vi "Main - UDP.vi"() -> ()   [LabVIEW 2023]
uses:
  <vilib>/addons/VeriStand Custom Device Scripting APIs/Data Sharing Framework/DSF Core.lvlibp/Typedefs/DSF Engine Framework Configuration.ctl
  <vilib>/addons/VeriStand Custom Device Scripting APIs/Data Sharing Framework/DSF Core.lvlibp/Typedefs/DSF Engine Plugin Configuration.ctl
  <vilib>/addons/VeriStand Custom Device Scripting APIs/Data Sharing Framework/DSF Core.lvlibp/Typedefs/Core Plugin Configuration.ctl
  <vilib>/addons/VeriStand Custom Device Scripting APIs/Data Sharing Framework/DSF Core.lvlibp/Typedefs/DSF Timing Info.ctl
  <vilib>/addons/VeriStand Custom Device Scripting APIs/Data Sharing Framework/DSF Core.lvlibp/Typedefs/DSF Settings Info.ctl
  <vilib>/addons/VeriStand Custom Device Scripting APIs/Data Sharing Framework/DSF Core.lvlibp/Typedefs/DSF Engine Plugin Thread Configuration.ctl
  <vilib>/addons/VeriStand Custom Device Scripting APIs/Data Sharing Framework/DSF Core.lvlibp/Typedefs/Core Thread Configuration.ctl
  <vilib>/addons/VeriStand Custom Device Scripting APIs/Data Sharing Framework/DSF Core.lvlibp/Typedefs/DSF Engine Transfer Group Configuration.ctl
  <vilib>/addons/VeriStand Custom Device Scripting APIs/Data Sharing Framework/DSF Core.lvlibp/Typedefs/Core Group Configuration.ctl
  <vilib>/addons/VeriStand Custom Device Scripting APIs/Data Sharing Framework/DSF Core.lvlibp/Typedefs/DSF Direction.ctl
  <vilib>/addons/VeriStand Custom Device Scripting APIs/Data Sharing Framework/DSF Core.lvlibp/Typedefs/DSF Timeout Behavior.ctl
  <vilib>/addons/VeriStand Custom Device Scripting APIs/Data Sharing Framework/DSF Core.lvlibp/Typedefs/DSF Engine Transfer Configuration.ctl
  <vilib>/addons/VeriStand Custom Device Scripting APIs/Data Sharing Framework/DSF Core.lvlibp/Typedefs/Core Transfer Configuration.ctl
  <vilib>/addons/VeriStand Custom Device Scripting APIs/Data Sharing Framework/DSF Core.lvlibp/Typedefs/DSF Engine Channel Configuration.ctl
  <vilib>/addons/VeriStand Custom Device Scripting APIs/Data Sharing Framework/DSF Core.lvlibp/Typedefs/Core Channel Configuration.ctl
  <vilib>/addons/VeriStand Custom Device Scripting APIs/Data Sharing Framework/DSF Core.lvlibp/Typedefs/DSF Data Type.ctl
  <userlib>/_OpenG.lib/array/array.llb/Index 1D Array Elements (String)__ogtk.vi
  <userlib>/_OpenG.lib/array/array.llb/Remove Duplicates from 1D Array (String)__ogtk.vi
  <userlib>/_OpenG.lib/array/array.llb/Filter 1D Array with Scalar (String)__ogtk.vi
  <vilib>/addons/VeriStand Custom Device Scripting APIs/Data Sharing Framework/DSF Core.lvlibp
  <vilib>/addons/VeriStand Custom Device Scripting APIs/Data Sharing Framework/DSF Core.lvlibp/Classes/Configuration/Core/Channel/Channel Configuration.lvclass
  <userlib>/_OpenG.lib/array/array.llb/openg_array.lvlib
  <vilib>/addons/VeriStand Custom Device Scripting APIs/Data Sharing Framework/DSF Core.lvlibp/Classes/Configuration/Core/Plugin/Plugin Configuration.lvclass
  <vilib>/addons/VeriStand Custom Device Scripting APIs/Data Sharing Framework/DSF Core.lvlibp/Classes/Configuration/Core/Thread/Thread Configuration.lvclass
  <vilib>/addons/VeriStand Custom Device Scripting APIs/Data Sharing Framework/DSF Core.lvlibp/Classes/Configuration/Core/Group/Group Configuration.lvclass
  <vilib>/addons/VeriStand Custom Device Scripting APIs/Data Sharing Framework/DSF Core.lvlibp/Classes/Configuration/Core/Transfer/Transfer Configuration.lvclass
panel:
  in  "Tab Control":enum32{"Main", "Raw Data", "Raw JSON"}(tab)
  out "DSF Clusters":T1[](array[typedef])
  out "Target Sources":string[](array[string])
  out "Channel Names":string[](array[string])
  out "Channel Units":string[](array[string])
  out "Channel Types":string[](array[string])
  out "Target Destinations":string[][](array[string])
  out "JSON Strings":string[](array[string])
  out "IP Addresses":string[](array[string])
  out "Target Names":string[](array[string])
  in  "File Path Control":path
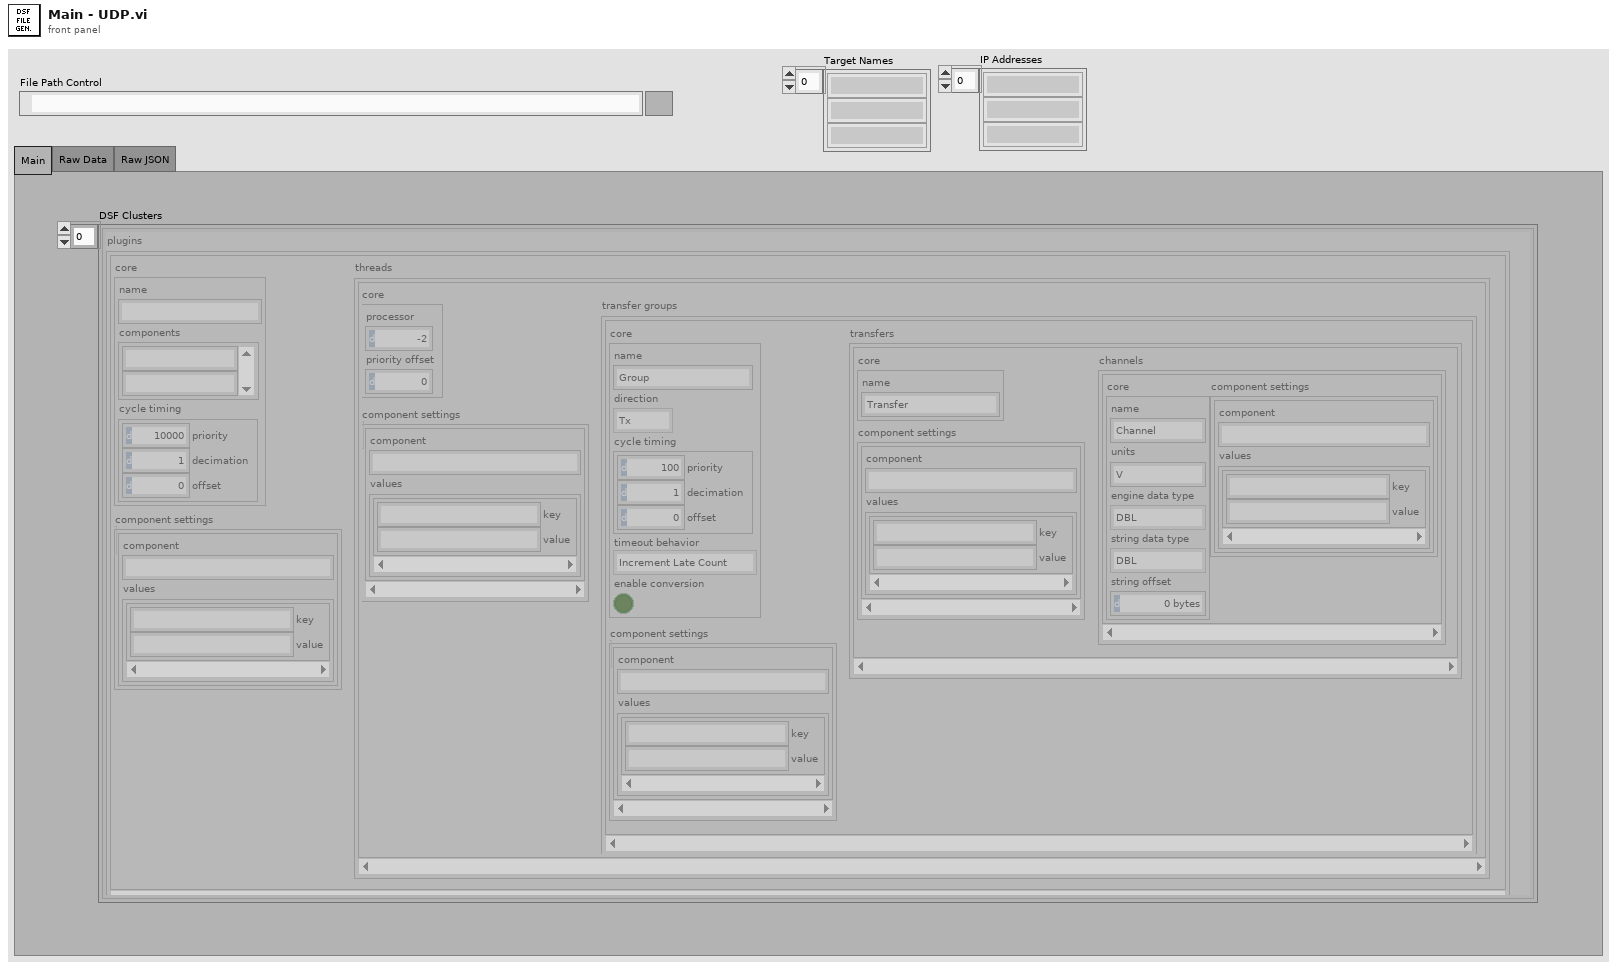
[diagram p1: front panel]
types:
  T1 = typedef "DSF Core.lvlibp/DSF Engine Framework Configuration.ctl" = cluster{"plugins":T2[]}
  T2 = typedef "DSF Core.lvlibp/DSF Engine Plugin Configuration.ctl" = cluster{"core":T3, "component settings":T5[], "threads":T6[]}
  T3 = typedef "DSF Core.lvlibp/Plugin Configuration.lvclass/Core Plugin Configuration.ctl" = cluster{"name":string, "components":string[], "cycle timing":T4}
  T4 = typedef "DSF Core.lvlibp/DSF Timing Info.ctl" = cluster{"priority":u64, "decimation":u64, "offset":u64}
  T5 = typedef "DSF Core.lvlibp/DSF Settings Info.ctl" = cluster{"component":string, "values":cluster{"key":string, "value":string}[]}
  T6 = typedef "DSF Core.lvlibp/DSF Engine Plugin Thread Configuration.ctl" = cluster{"core":T7, "component settings":T5[], "transfer groups":T8[]}
  T7 = typedef "DSF Core.lvlibp/Thread Configuration.lvclass/Core Thread Configuration.ctl" = cluster{"processor":i32, "priority offset":i16}
  T8 = typedef "DSF Core.lvlibp/DSF Engine Transfer Group Configuration.ctl" = cluster{"core":T9, "component settings":T5[], "transfers":T12[]}
  T9 = typedef "DSF Core.lvlibp/Group Configuration.lvclass/Core Group Configuration.ctl" = cluster{"name":string, "direction":T10, "cycle timing":T4, "timeout behavior":T11, "enable conversion":bool}
  T10 = typedef "DSF Core.lvlibp/DSF Direction.ctl" = enum8{"Tx", "Rx"}
  T11 = typedef "DSF Core.lvlibp/DSF Timeout Behavior.ctl" = enum8{"Increment Late Count", "Throw Error"}
  T12 = typedef "DSF Core.lvlibp/DSF Engine Transfer Configuration.ctl" = cluster{"core":T13, "component settings":T5[], "channels":T14[]}
  T13 = typedef "DSF Core.lvlibp/Transfer Configuration.lvclass/Core Transfer Configuration.ctl" = cluster{"name":string}
  T14 = typedef "DSF Core.lvlibp/DSF Engine Channel Configuration.ctl" = cluster{"core":T15, "component settings":T5[]}
  T15 = typedef "DSF Core.lvlibp/Channel Configuration.lvclass/Core Channel Configuration.ctl" = cluster{"name":string, "units":string, "engine data type":T16, "string data type":T16, "string offset":u64}
  T16 = typedef "DSF Core.lvlibp/DSF Data Type.ctl" = enum8{"Bool", "SGL", "DBL", "I8", "I16", "I32", "I64", "U8", "U16", "U32", "U64"}
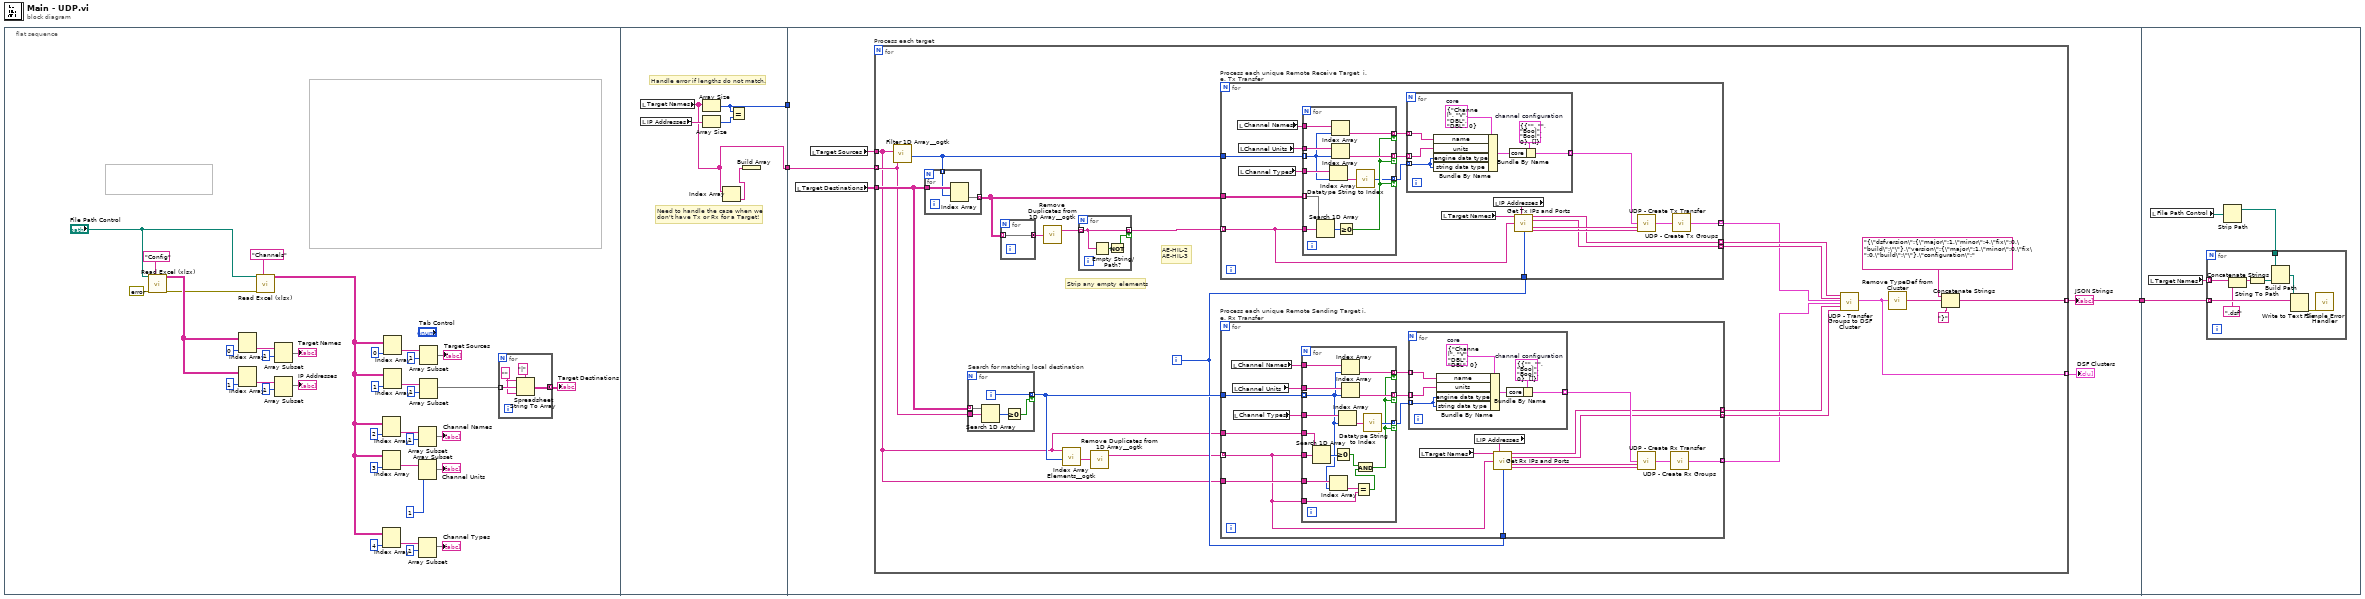
[diagram p0: block diagram]
diagram:
  n1 = flat-sequence {
    tunnel: [w47] -> w3
    tunnel: [w44] -> w1
    tunnel: w3 -> [_]
    tunnel: [w49] -> w2
    tunnel: w1 -> [w53]
    tunnel: w2 -> [w173]
    frame #0 {
      n2 = call "Read Excel (xlsx).vi"("Excel._SheetName"="Config", "error in (no error)"=errorcluster {"status"=FALSE, "code"=0, "source"=""}, "File Path Control"="File Path Control") -> ("error out"=w9:errorcluster, "data"=w10:string[][])  [unwired: 7 in]
      n3 = Index Array(array=w10, index (col)=0 ("disabled index (col)")) -> (element=w37:string[])  [unwired: 1 in]
      n4 = Index Array(array=w10, index (col)=1 ("disabled index (col)")) -> (element=w33:string[])  [unwired: 1 in]
      n5 = call "Read Excel (xlsx).vi"("Excel._SheetName"="Channels", "error in (no error)"=w9, "File Path Control"="File Path Control") -> ("data"=w8:string[][])  [unwired: 7 in, 1 out]
      n6 = Array Subset(array=w37, index=1) -> (→"Target Names":string[])  [unwired: 1 in]
      n7 = Array Subset(array=w33, index=1) -> (→"IP Addresses":string[])  [unwired: 1 in]
      n8 = Index Array(array=w8, index (col)=2 ("disabled index (col)")) -> (element=w22:string[])  [unwired: 1 in]
      n9 = Index Array(array=w8, index (col)=3 ("disabled index (col)")) -> (element=w18:string[])  [unwired: 1 in]
      n10 = Index Array(array=w8, index (col)=4 ("disabled index (col)")) -> (element=w14:string[])  [unwired: 1 in]
      n11 = Index Array(array=w8, index (col)=0 ("disabled index (col)")) -> (element=w29:string[])  [unwired: 1 in]
      n12 = Index Array(array=w8, index (col)=1 ("disabled index (col)")) -> (element=w25:string[])  [unwired: 1 in]
      n13 = Array Subset(array=w22, index=1) -> (→"Channel Names":string[])  [unwired: 1 in]
      n14 = Array Subset(array=w18, index=1) -> (→"Channel Units":string[])  [unwired: 1 in]
      n15 = Array Subset(array=w14, index=1) -> (→"Channel Types":string[])  [unwired: 1 in]
      n16 = Array Subset(array=w29, index=1) -> (→"Target Sources":string[])  [unwired: 1 in]
      n17 = Array Subset(array=w25, index=1) -> (w5:string[])  [unwired: 1 in]
      n18 = for {
        tunnel: w5 -> [w43] mode=indexing
        tunnel: [w41] -> w4 mode=concatenating
        w40 = ""
        n19 = Spreadsheet String To Array(delimiter (Tab)="|", format string=w40, spreadsheet string=w43, array type (2D Dbl)=w40) -> (array=w41:string[][])
      }
      "Target Destinations" <- w4
    }
    frame #1 {
      # "Need to handle the case when we \ndon't have Tx or Rx for a Target!"
      # "Handle error if lengths do not match."
      n20 = local read "Target Names"() -> (w44:string[])
      n21 = local read "IP Addresses"() -> (w46:string[])
      n22 = Array Size(array=w44) -> (size(s)=w47:i32)
      n23 = Array Size(array=w46) -> (size(s)=w48:i32)
      n24 = Index Array(array=w44) -> (element=w45:string)  [unwired: 1 in]
      n25 = Equal?(x=w47, y=w48) -> ()  [unwired: 1 out]
      n26 = Build Array(w45) -> ()  [unwired: 1 out]
    }
    frame #2 {
      n27 = local read "Target Destinations"() -> (w51:string[][])
      n28 = local read "Target Sources"() -> (w52:string[])
      n29 = for "Process each target" {
        tunnel: w53 -> [w61] mode=indexing
        tunnel: w52 -> [w60]
        tunnel: w51 -> [w70]
        tunnel: [w64] -> w49 mode=indexing
        tunnel: [w63] -> w50 mode=indexing
        i -> [w68]
        # "AE-HIL-2\nAE-HIL-3"
        # "Strip any empty elements"
        n30 = call-poly <userlib>:"Filter 1D Array__ogtk.vi"("items to filter"=w61, "array"=w60) -> ("filtered item indices"=w73:i32[])  [unwired: 4 in, 1 out]
        n31 = for {
          tunnel: w73 -> [w169] mode=indexing
          tunnel: w70 -> [w170]
          tunnel: [w168] -> w72 mode=indexing
          n32 = Index Array(array=w170, index (row)=w169) -> (element=w168:string[])  [unwired: 1 in]
        }
        n33 = for "Search for matching local destination" {
          tunnel: w70 -> [w125] mode=indexing
          tunnel: w61 -> [w124]
          tunnel: [w122] -> w69 mode=indexing if=w121
          i -> [w122]
          n34 = Search 1D Array(1D array=w125, element=w124) -> (index of element=w123:i32)  [unwired: 1 in]
          n35 = Greater Or Equal To 0?(x=w123) -> (x >= 0?=w121:bool)
        }
        n36 = for {
          tunnel: w72 -> [w167] mode=indexing
          tunnel: [w167] -> w76 mode=concatenating
        }
        n37 = call-poly <userlib>:"Remove Duplicates from 1D Array__ogtk.vi"("Input Array"=w76) -> ("Output Array"=w75:string[])  [unwired: 1 out]
        n38 = call-poly <userlib>:"Index Array Elements__ogtk.vi"("indices"=w69, "array"=w60) -> ("elements"=w71:string[])  [unwired: 9 in]
        n39 = for {
          tunnel: w75 -> [w166] mode=indexing
          tunnel: [w166] -> w74 mode=indexing if=w164
          n40 = Empty String/Path?(string/path=w166) -> (empty?=w165:bool)
          n41 = Not(x=w165) -> (.not. x?=w164:bool)
        }
        n42 = call-poly <userlib>:"Remove Duplicates from 1D Array__ogtk.vi"("Input Array"=w71) -> ("Output Array"=w62:string[])  [unwired: 1 out]
        n43 = for "Process each unique Remote Receive Target  i.e. Tx Transfer" {
          tunnel: w74 -> [w134] mode=indexing
          tunnel: w73 -> [w144]
          tunnel: w72 -> [w143]
          tunnel: w68 -> [w135]
          tunnel: [w131] -> w59 mode=indexing
          tunnel: [w130] -> w58 mode=indexing
          tunnel: [w126] -> w55 mode=indexing
          n44 = local read "Channel Names"() -> (w142:string[])
          n45 = local read "Channel Units"() -> (w141:string[])
          n46 = local read "Channel Types"() -> (w129:string[])
          n47 = for {
            tunnel: w143 -> [w163] mode=indexing
            tunnel: w134 -> [w162]
            tunnel: w144 -> [w155] mode=indexing
            tunnel: w142 -> [w160]
            tunnel: w141 -> [w159]
            tunnel: [w158] -> w140 mode=indexing if=w154
            tunnel: [w157] -> w139 mode=indexing if=w154
            tunnel: w129 -> [w156]
            tunnel: [w152] -> w128 mode=indexing if=w154
            n48 = Search 1D Array(1D array=w163, element=w162) -> (index of element=w161:i32)  [unwired: 1 in]
            n49 = Index Array(array=w156, index=w155) -> (element=w153:string)
            n50 = Index Array(array=w160, index=w155) -> (element=w158:string)
            n51 = Index Array(array=w159, index=w155) -> (element=w157:string)
            n52 = Greater Or Equal To 0?(x=w161) -> (x >= 0?=w154:bool)
            n53 = call "Datatype String to Index.vi"("Datatype String"=w153) -> ("Datatype"=w152:T16)  [unwired: 14 in]
          }
          n54 = for {
            tunnel: w140 -> [w148] mode=indexing
            tunnel: w139 -> [w147] mode=indexing
            tunnel: [w146] -> w138 mode=indexing
            tunnel: w128 -> [w145] mode=indexing
            w149 = T15 {"name"="Channel", "units"="V", "engine data type"=enum."DBL", "string data type"=enum."DBL", "string offset"=0}  # core
            w150 = T14 {"core"={"name"="", "units"="", "engine data type"=enum."Bool", "string data type"=enum."Bool", "string offset"=0}, "component settings"=[]}  # channel configuration
            n55 = Bundle By Name(cluster=w149, "name"=w148, "units"=w147, "engine data type"=w145, "string data type"=w145) -> (w151:T15)
            n56 = Bundle By Name(cluster=w150, "core"=w151) -> (w146:T14)
          }
          n57 = local read "Target Names"() -> (w132:string[])
          n58 = local read "IP Addresses"() -> (w133:string[])
          n59 = call "Get Tx IPs and Ports.vi"("Target Names"=w132, "IP Addresses"=w133, "Remote Target Name"=w134, "Local Target Index"=w135) -> ("Local IP Address"=w131:string, "Local Port Number"=w130:string, "Remote IP Address"=w137:string, "Remote Port Number"=w136:string)  [unwired: 8 in]
          n60 = call "UDP - Create Tx Transfer.vi"("tx channels"=w138, "destination address"=w137, "destination port"=w136) -> ("Transfer"=w127:T12)  [unwired: 12 in]
          n61 = call "UDP - Create Tx Groups.vi"("Tx Transfers"=w127) -> ("Tx Transfer Group"=w126:T8)  [unwired: 14 in]
        }
        n62 = for "Process each unique Remote Sending Target i.e. Rx Transfer" {
          tunnel: w62 -> [w85] mode=indexing
          tunnel: w69 -> [w96]
          tunnel: w60 -> [w95]
          tunnel: w68 -> [w89]
          tunnel: w60 -> [w86]
          tunnel: [w84] -> w57 mode=indexing
          tunnel: [w83] -> w56 mode=indexing
          tunnel: [w78] -> w54 mode=indexing
          n63 = local read "Channel Names"() -> (w94:string[])
          n64 = local read "Channel Units"() -> (w93:string[])
          n65 = local read "Channel Types"() -> (w79:string[])
          n66 = for {
            tunnel: w85 -> [w119]
            tunnel: w96 -> [w104] mode=indexing
            tunnel: w95 -> [w108]
            tunnel: w94 -> [w118]
            tunnel: w93 -> [w117]
            tunnel: [w116] -> w92 mode=indexing if=w106
            tunnel: [w115] -> w91 mode=indexing if=w106
            tunnel: w86 -> [w114]
            tunnel: w85 -> [w112]
            tunnel: [w107] -> w80 mode=indexing if=w106
            tunnel: w79 -> [w105]
            n67 = Search 1D Array(1D array=w108, element=w119) -> (index of element=w120:i32)  [unwired: 1 in]
            n68 = Index Array(array=w114, index=w104) -> (element=w113:string)
            n69 = Greater Or Equal To 0?(x=w120) -> (x >= 0?=w111:bool)
            n70 = Index Array(array=w105, index=w104) -> (element=w109:string)
            n71 = Index Array(array=w118, index=w104) -> (element=w116:string)
            n72 = Index Array(array=w117, index=w104) -> (element=w115:string)
            n73 = Equal?(x=w113, y=w112) -> (x = y?=w110:bool)
            n74 = And(x=w111, y=w110) -> (x .and. y?=w106:bool)
            n75 = call "Datatype String to Index.vi"("Datatype String"=w109) -> ("Datatype"=w107:T16)  [unwired: 14 in]
          }
          n76 = for {
            tunnel: w92 -> [w100] mode=indexing
            tunnel: w91 -> [w99] mode=indexing
            tunnel: [w98] -> w90 mode=indexing
            tunnel: w80 -> [w97] mode=indexing
            w101 = T15 {"name"="Channel", "units"="V", "engine data type"=enum."DBL", "string data type"=enum."DBL", "string offset"=0}  # core
            w102 = T14 {"core"={"name"="", "units"="", "engine data type"=enum."Bool", "string data type"=enum."Bool", "string offset"=0}, "component settings"=[]}  # channel configuration
            n77 = Bundle By Name(cluster=w101, "name"=w100, "units"=w99, "engine data type"=w97, "string data type"=w97) -> (w103:T15)
            n78 = Bundle By Name(cluster=w102, "core"=w103) -> (w98:T14)
          }
          n79 = local read "Target Names"() -> (w87:string[])
          n80 = local read "IP Addresses"() -> (w88:string[])
          n81 = call "Get Rx IPs and Ports.vi"("Target Names"=w87, "IP Addresses"=w88, "Remote Target Name"=w85, "Local Target Index"=w89) -> ("Local IP Address"=w84:string, "Local Port Number"=w83:string, "Remote IP Address"=w82:string, "Remote Port Number"=w81:string)  [unwired: 8 in]
          n82 = call "UDP - Create Rx Transfer.vi"("rx channels"=w90, "source address"=w82, "source port"=w81) -> ("Transfer"=w77:T12)  [unwired: 12 in]
          n83 = call "UDP - Create Rx Groups.vi"("Rx Transfers"=w77) -> ("Rx Transfer Group"=w78:T8)  [unwired: 14 in]
        }
        n84 = call "UDP - Transfer Groups to DSF Cluster.vi"("Tx local address"=w59, "Tx local port"=w58, "Tx Transfer Groups"=w55, "Rx Transfer Groups"=w54, "Rx local address"=w57, "Rx local port"=w56) -> ("DSF Cluster"=w63:T1)  [unwired: 13 in]
        n85 = call "Remove TypeDef from Cluster.vi"("configuration 1.4"=w63) -> ("JSON string"=w67:string)  [unwired: 14 in]
        n86 = Concatenate Strings("{\"dsfversion\":{\"major\":1,\"minor\":4,\"fix\":0,\"build\":\"\"},\"version\":{\"major\":1,\"minor\":0,\"fix\":0,\"build\":\"\"},\"configuration\":", w67, "}") -> (w64:string)
      }
      "JSON Strings" <- w49
      "DSF Clusters" <- w50
    }
    frame #3 {
      n87 = local read "Target Names"() -> (w172:string[])
      n88 = local read "File Path Control"() -> (w174:path)
      n89 = Strip Path(path=w174) -> (stripped path=w171:path)  [unwired: 1 out]
      n90 = for {
        tunnel: w173 -> [w182] mode=indexing
        tunnel: w172 -> [w178] mode=indexing
        tunnel: w171 -> [w181]
        n91 = Concatenate Strings(w178, ".dsf" ("string")) -> (w177:string)
        n92 = String To Path(string=w177) -> (path=w180:path)
        n93 = Build Path(base path=w181, name or relative path=w180) -> (appended path=w179:path)
        n94 = Write to Text File(file (use dialog)=w179, text=w182) -> (error out=w175:errorcluster)  [unwired: 2 in, 2 out]
        n95 = call <vilib>:"Simple Error Handler.vi"("error in (no error)"=w175) -> ()  [unwired: 4 in, 5 out]
      }
    }
  }
